vi "rs3 get stream profile 2.vi"(8 "error in (no error)":errorcluster, 10 "index":i32, 11 "Stream Profile list in":u64) -> (0 "error out":errorcluster, 1 "stream profile":u64, 2 "error out":u64, 3 "Stream Profile list out":u64)   [LabVIEW 2018, in "libRealSense3.lvlib"]
doc: "Block until new frames are available. This must be called before calling Get Frame Data. \n\nOutput\nerror if non-null, receives any error that occurs during this call, otherwise, errors are ignored"
uses:
  libRealSense3.lvlib
  realsense2.dll
panel:
  # "RS3 Get Stream Profile"
  # "(C) Intel Corp.,  AGJ 2017"
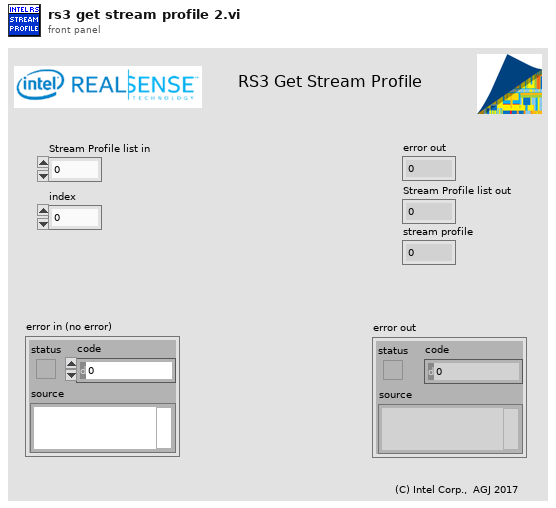
[diagram p1: front panel]
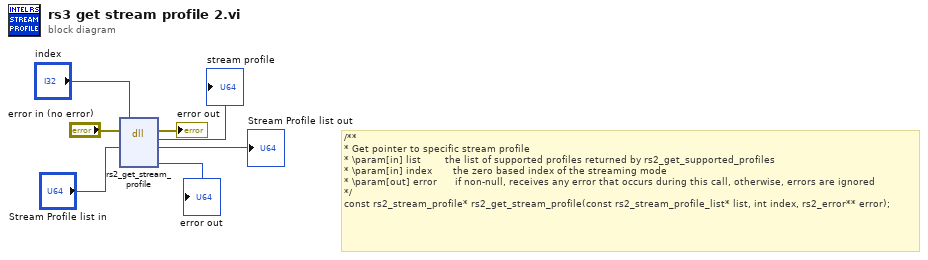
[diagram p0: block diagram]
diagram:
  # "/**\n* Get pointer to specific stream profile\n* \\param[in] list        the list of supported profiles returned by rs2_get_supported_profiles\n* \\param[in] index       the zero based index of the streaming mode\n* \\param[out] error      if non-null, receives any error that occurs during this call, otherwise, errors are ignored\n*/\nconst rs2_stream_profile* rs2_get_stream_profile(const rs2_stream_profile_list* list, int index, rs2_error** error);"
  n1 = dll-call lib="C:/Users/aaron.jencks/Documents/Temp/realsense_labview_sdk/RealSense SDK2.11.0 for LabVIEW/realsense2.dll" fn="rs2_get_stream_profile"(error in="error in (no error)", "stream profile list"="Stream Profile list in", "index"="index") -> (error out=→"error out":errorcluster, "stream profile"=→"stream profile":u64, "stream profile list"=→"Stream Profile list out":u64, "error"=→"error out":u64)  [unwired: 4 in, 1 out]
